vi "setVel.vi"(2 "error in (no error)":errorcluster, 3 "speed":dbl=0.5 min=0.5 max=2.1 step=0.1, 4 "UART in":refnum<visa-resource-name>) -> (0 "error out":errorcluster, 1 "UART out":refnum<visa-resource-name>)   [LabVIEW 2016]
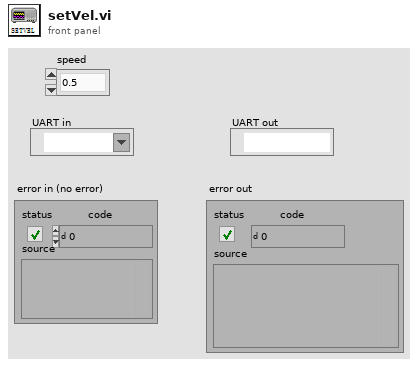
[diagram p1: front panel]
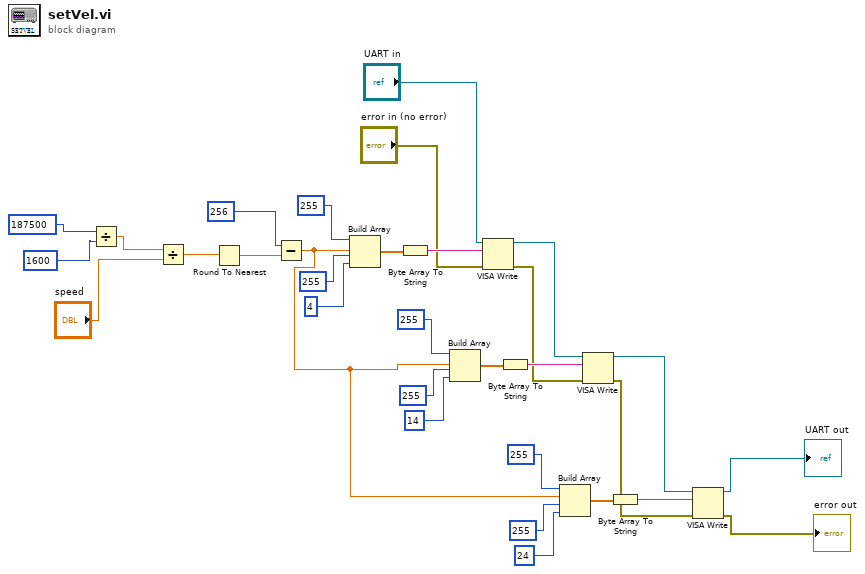
[diagram p0: block diagram]
diagram:
  n1 = Divide(x=187500, y=1600) -> (x/y=w29:dbl)
  n2 = Divide(x=w29, y="speed") -> (x/y=w27:dbl)
  n3 = Round To Nearest(number=w27) -> (nearest integer value=w26:dbl)
  n4 = Subtract(x=256, y=w26) -> (x-y=w9:dbl)
  n5 = Build Array(255, w9, 255, 4) -> (w21:dbl[])
  n6 = Byte Array To String(unsigned byte array=w21) -> (string=w20:string)
  n7 = Build Array(255, w9, 255, 14) -> (w16:dbl[])
  n8 = VISA Write(VISA resource name="UART in", write buffer=w20, error in (no error)="error in (no error)") -> (VISA resource name out=w6:refnum<visa-resource-name>, error out=w5:errorcluster)  [unwired: 1 out]
  n9 = Byte Array To String(unsigned byte array=w16) -> (string=w15:string)
  n10 = Build Array(255, w9, 255, 24) -> (w11:dbl[])
  n11 = VISA Write(VISA resource name=w6, write buffer=w15, error in (no error)=w5) -> (VISA resource name out=w4:refnum<visa-resource-name>, error out=w3:errorcluster)  [unwired: 1 out]
  n12 = Byte Array To String(unsigned byte array=w11) -> (string=w10:string)
  n13 = VISA Write(VISA resource name=w4, write buffer=w10, error in (no error)=w3) -> (VISA resource name out=→"UART out":refnum<visa-resource-name>, error out=→"error out":errorcluster)  [unwired: 1 out]
